vi "Get Analog AO DAQ Node.vi"(0 "DAQ":refnum<class "DAQ.lvclass">, 5 "IOName (enum)":variant, 9 "Name":string, 11 "error in (no error)":errorcluster) -> (4 "DAQ":refnum<class "DAQ.lvclass">, 8 "AO DAQNode out":T1 {"Conversion"."ScaleOffset" format="%.3f"; "Conversion"."MinEngUnit" format="%.3f"; "Conversion"."MaxEngUnit" format="%.3f"; "Conversion"."MinSignal" format="%.3f"; "Conversion"."MaxSignal" format="%.3f"}, 15 "error out":errorcluster)   [LabVIEW 2017, in "DAQ.lvclass"]
doc: "Developed by Kevin Thompson\nkevin@thompsonengineering.net\n\nCopyright 2018-2020\nThompson Engineering, LLC"
uses:
  DAQ.lvclass
  DataTypes/TD AO Channel--cluster.ctl
  DataTypes/TD DataValueConversion--cluster.ctl
  DAQ.lvclass/DAQ.ctl
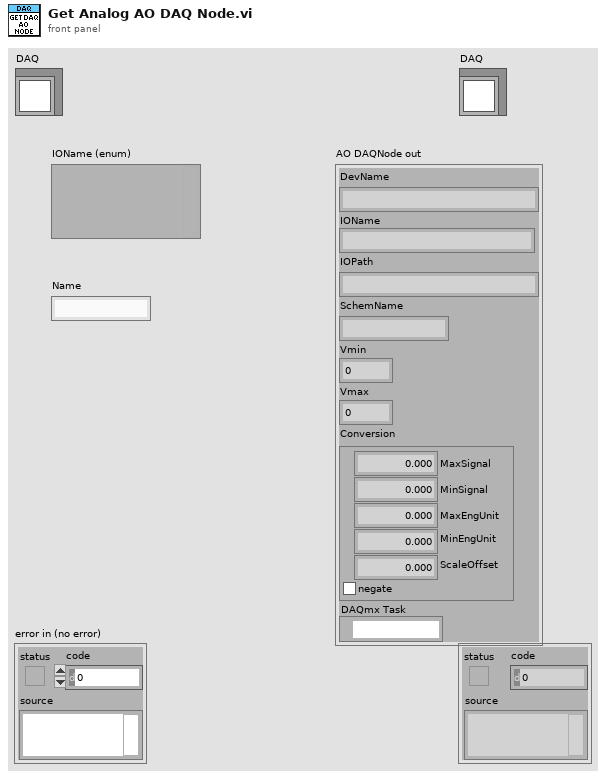
[diagram p1: front panel]
types:
  T1 = typedef "DAQ.lvclass/TD AO Channel--cluster.ctl" = cluster{"DevName":string, "IOName":string, "IOPath":string, "SchemName":string, "Vmin":dbl, "Vmax":dbl, "Conversion":T2, "DAQmx Task":refnum<k21>}
  T2 = typedef "DAQ.lvclass/TD DataValueConversion--cluster.ctl" = cluster{"MaxSignal":dbl, "MinSignal":dbl, "MaxEngUnit":dbl, "MinEngUnit":dbl, "ScaleOffset":dbl, "negate":bool}
  T3 = typedef "Type Descriptor Enumeration__ogtk.ctl" = enum8{"<Null>", "I8", "I16", "I32", "I64", "U8", "U16", "U32", "U64", "SGL", "DBL", "EXT", "CSG", "CDB", "CXT", "0x0F", "0x10", "0x11", "0x12", "0x13", "0x14", "Enum U8", "Enum U16", "Enum U32", "Enum U64", "SGL PQ", "DBL PQ", "EXT PQ", "CSG PQ", "CDB PQ", "CXT PQ", "0x1F", "0x20", "Boolean", "0x22", "0x23", "0x24", "0x25", "0x26", "0x27", "0x28", "0x29", "0x2A", "0x2B", "0x2C", "0x2D", "0x2E", "0x2F", "String", "0x31", "Path", "Pict", "0x34", "0x35", "0x36", "DAQ", "0x38", "0x39", "0x3A", "0x3B", "0x3C", "0x3D", "0x3E", "0x3F", "Array", "0x41", "0x42", "0x43", "0x44", "0x45", "0x46", "0x47", "0x48", "0x49", "0x4A", "0x4B", "0x4C", "0x4D", "0x4E", "0x4F", "Cluster", "0x51", "0x52", "Variant", "Waveform", "0x55", "0x56", "0x57", "0x58", "0x59", "0x5A", "0x5B", "0x5C", "0x5D", "0x5E", "0x5F", "0x60", "0x61", "0x62", "0x63", "0x64", "0x65", "0x66", "0x67", "0x68", "0x69", "0x6A", "0x6B", "0x6C", "0x6D", "0x6E", "0x6F", "Refnum"}
  T4 = typedef "TD Dynamic CVT DVR--ref.ctl" = refnum<data-value>
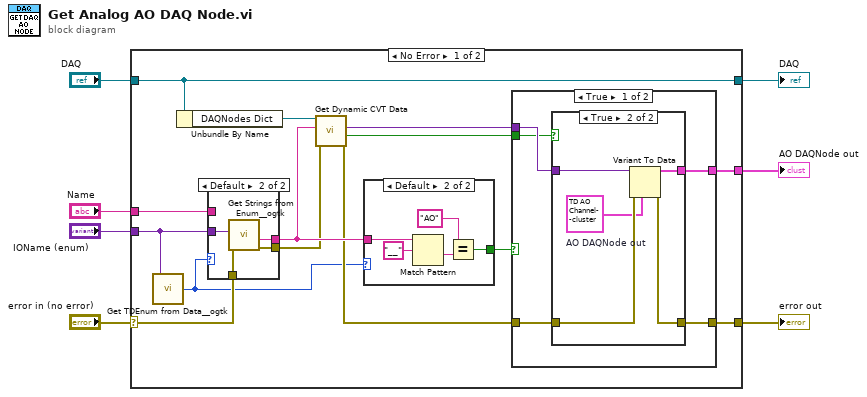
[diagram p0: block diagram]
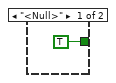
[diagram p2: hidden frame]
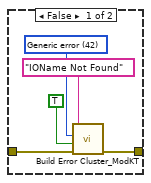
[diagram p4: hidden frame]
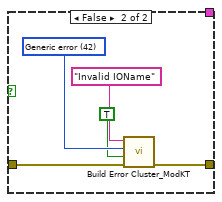
[diagram p5: hidden frame]
diagram:
  n1 = case shown="No Error" "error in (no error)" {
    selector: "error in (no error)" -> [w21 w55]
    tunnel: [w15 w55] -> w6
    tunnel: [w20 w54] -> w4
    tunnel: "DAQ" -> [w20 w54]
    tunnel: "IOName (enum)" -> [w11 _]
    tunnel: [w12 _] -> w2
    tunnel: "Name" -> [w9 _]
    frame No Error {
      n2 = call <userlib>:"Get TDEnum from Data__ogtk.vi"("Data"=w11) -> ("Type Descriptor Enumeration"=w10:T3)  [unwired: 4 in]
      n3 = Unbundle By Name(w20) -> ("DAQNodes Dict"=w19:T4)
      n4 = case shown="Default" w10 {
        tunnel: w21 -> [w28 w33]
        tunnel: [w29 w32] -> w18
        tunnel: [w28 w31] -> w17
        tunnel: w11 -> [_ w30]
        tunnel: w9 -> [w29 _]
        frame "<Null>" {
        }
        frame Default {
          n5 = call <userlib>:"Get Strings from Enum__ogtk.vi"("error in (no error)"=w33, "Enum"=w30) -> ("error out"=w31:errorcluster, "String Value"=w32:string)  [unwired: 6 in, 2 out]
        }
      }
      n6 = call <vilib>:"Get Dynamic CVT Data.vi"("error in (no error)"=w17, "DataName"=w18, "dCVT DVR"=w19) -> ("error out"=w16:errorcluster, "found"=w13:bool, "value"=w14:variant)  [unwired: 5 in, 1 out]
      n7 = case shown="Default" w10 {
        tunnel: w18 -> [_ w27]
        tunnel: [TRUE w23] -> w8
        frame "<Null>" {
        }
        frame Default {
          n8 = Match Pattern(string=w27, regular expression="__") -> (after substring=w25:string)  [unwired: 1 in, 3 out]
          n9 = Equal?(x="AO", y=w25) -> (x = y?=w23:bool)
        }
      }
      n10 = case shown="True" w8 {
        tunnel: w16 -> [w38 w52]
        tunnel: [w37 w53] -> w15
        tunnel: w14 -> [w36 _]
        tunnel: w13 -> [w34 _]
        tunnel: [w35 _] -> w12
        frame True {
          n11 = case shown="True" w34 {
            tunnel: w38 -> [w40 w48]
            tunnel: [w39 w47] -> w37
            tunnel: w36 -> [_ w46]
            tunnel: [_ w45] -> w35
            frame False {
              w42 = 42 items=["No error", "Argument error", "Memory is full", "Out of zone", "End of file", "File already open", "Generic file I/O error", "File not found", "File permission error", "Disk is full", "Duplicate path", "Too many files open", "System feature not enabled", "Resource file not found", "Cannot add resource", "Resource not found", "Image not found", "Image memory error", "Pen does not exist", "Config type invalid", "Config token not found", "Config parse error", "Config memory error", "Bad external code format", "Bad external code offset", "External code not present", "Null window", "Destroy window error", "Null menu", "Print aborted", "Bad print record", "Print driver error", "Windows error during printing", "Memory error during printing", "Print dialog error", "Generic print error", "Invalid device refnum", "Device not found", "Device parameter error", "Device unit error", "Cannot open device", "Device call aborted", "Generic error", "Cancelled by user", "Object ID too low", "Object ID too high", "Object not in heap", "Unknown heap", "Unknown object (invalid DefProc)", "Unknown object (DefProc not in table)", "Message out of range", "Invalid (null) method", "Unknown message", "Manager call not supported", "Bad address", "Network operation in progress", "Network operation timed out", "Connection is busy", "Network attribute not supported", "Network error", "Address in use", "System out of memory", "Connection aborted", "Connection refused", "Not connected", "Already connected", "Connection closed", "Initialization error (interapplication manager)", "Bad occurrence", "Wait on unbound occurrence handler", "Occurrence queue overflow", "Datalog type conflict", "Unused", "Unrecognized type (interapplication manager)", "Memory corrupt", "Failed to make temporary DLL", "Old CIN version", "Drag socket not found", "Failed to load drop-object", "Failed to register OLE object", "Failed to release OLE object", "Format specifier type mismatch", "Unknown format specifier", "Too few format specifiers", "Too many format specifiers", "Scan failed", "Newer CIN version", "Error converting to variant", "Runtime menu error", "Password tampered", "Variant attribute not found", "Incompatible variant data type", "Event data is not available", "Event Store is not present", "Occurrence is not found", "Event Queue is not created", "Event info is not available", "Refnum passed is NULL", "Error retrieving Class GUID", "Error retrieving CoClass GUID", "Error retrieving TypeLib GUID.", "Bad built application magic bytes.", "Specific driver is different from the specific driver associated with the Logical Name.", "There is no session opened to the class driver.", "Max Error", "MAX - Error with config objects", "MAX - Error loading configuration", "MAX - Group not supported"]
              n12 = call <vilib>:"Build Error Cluster_ModKT .vi"("Prepend String (\"\")"="IOName Not Found" ("Prepend String (\"\")"), "code"=w42, "error? (F)"=TRUE, "error in (no error)"=w40) -> ("error out"=w39:errorcluster)  [unwired: 3 in, 1 out]
            }
            frame True {
              w44 = T1 {"DevName"="", "IOName"="", "IOPath"="", "SchemName"="", "Vmin"=0.0, "Vmax"=0.0, "Conversion"={"MaxSignal"=0.0, "MinSignal"=0.0, "MaxEngUnit"=0.0, "MinEngUnit"=0.0, "ScaleOffset"=0.0, "negate"=FALSE}, "DAQmx Task"=""}  # AO DAQNode out
              n13 = Variant To Data(error in=w48, type=w44, Variant=w46) -> (data=w45:T1, error out=w47:errorcluster)
            }
          }
        }
        frame False {
          w50 = 42 items=["No error", "Argument error", "Memory is full", "Out of zone", "End of file", "File already open", "Generic file I/O error", "File not found", "File permission error", "Disk is full", "Duplicate path", "Too many files open", "System feature not enabled", "Resource file not found", "Cannot add resource", "Resource not found", "Image not found", "Image memory error", "Pen does not exist", "Config type invalid", "Config token not found", "Config parse error", "Config memory error", "Bad external code format", "Bad external code offset", "External code not present", "Null window", "Destroy window error", "Null menu", "Print aborted", "Bad print record", "Print driver error", "Windows error during printing", "Memory error during printing", "Print dialog error", "Generic print error", "Invalid device refnum", "Device not found", "Device parameter error", "Device unit error", "Cannot open device", "Device call aborted", "Generic error", "Cancelled by user", "Object ID too low", "Object ID too high", "Object not in heap", "Unknown heap", "Unknown object (invalid DefProc)", "Unknown object (DefProc not in table)", "Message out of range", "Invalid (null) method", "Unknown message", "Manager call not supported", "Bad address", "Network operation in progress", "Network operation timed out", "Connection is busy", "Network attribute not supported", "Network error", "Address in use", "System out of memory", "Connection aborted", "Connection refused", "Not connected", "Already connected", "Connection closed", "Initialization error (interapplication manager)", "Bad occurrence", "Wait on unbound occurrence handler", "Occurrence queue overflow", "Datalog type conflict", "Unused", "Unrecognized type (interapplication manager)", "Memory corrupt", "Failed to make temporary DLL", "Old CIN version", "Drag socket not found", "Failed to load drop-object", "Failed to register OLE object", "Failed to release OLE object", "Format specifier type mismatch", "Unknown format specifier", "Too few format specifiers", "Too many format specifiers", "Scan failed", "Newer CIN version", "Error converting to variant", "Runtime menu error", "Password tampered", "Variant attribute not found", "Incompatible variant data type", "Event data is not available", "Event Store is not present", "Occurrence is not found", "Event Queue is not created", "Event info is not available", "Refnum passed is NULL", "Error retrieving Class GUID", "Error retrieving CoClass GUID", "Error retrieving TypeLib GUID.", "Bad built application magic bytes.", "Specific driver is different from the specific driver associated with the Logical Name.", "There is no session opened to the class driver.", "Max Error", "MAX - Error with config objects", "MAX - Error loading configuration", "MAX - Group not supported"]
          n14 = call <vilib>:"Build Error Cluster_ModKT .vi"("Prepend String (\"\")"="Invalid IOName" ("Prepend String (\"\")"), "code"=w50, "error? (F)"=TRUE, "error in (no error)"=w52) -> ("error out"=w53:errorcluster)  [unwired: 3 in, 1 out]
        }
      }
    }
    frame Error {
    }
  }
  "error out" <- w6
  "DAQ" <- w4
  "AO DAQNode out" <- w2
